vi "Apply Package Name to Enum Metadata.vi"(8 "error in":errorcluster, 10 "Package Name":string, 11 "gRPC Enum Metadata in":T1[](array[typedef])) -> (0 "error out":errorcluster, 3 "gRPC Enum Metadata out":T1[](array[typedef]))   [LabVIEW 2019, in "grpc-lvsupport.lvlib"]
uses:
  grpc-lvsupport.lvlib
  typeDefs/Enum Metadata.ctl
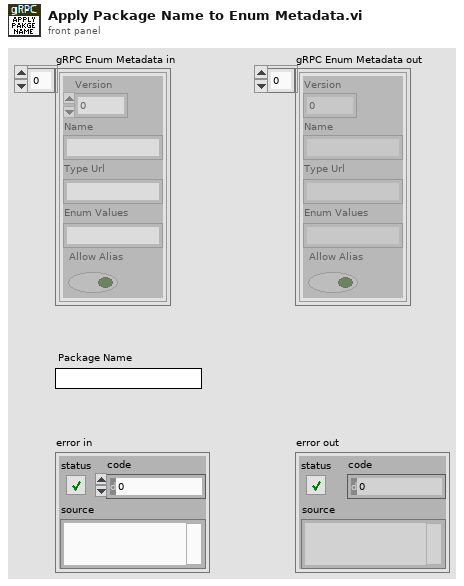
[diagram p1: front panel]
types:
  T1 = typedef "grpc-lvsupport.lvlib/Enum Metadata.ctl" = cluster{"Version":i32, "Name":string, "Type Url":string, "Enum Values":string, "Allow Alias":bool}
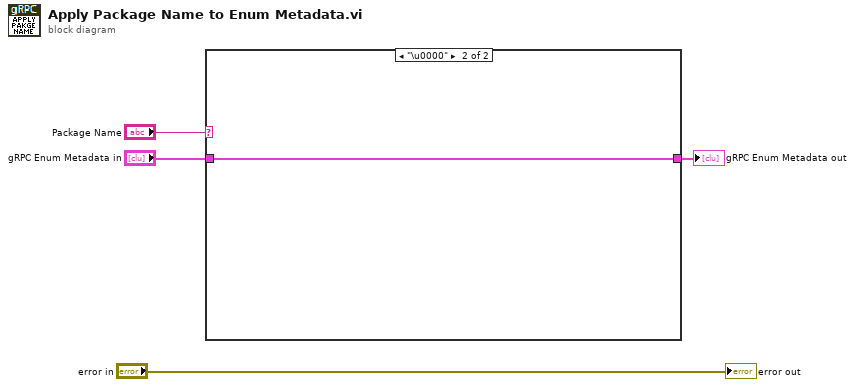
[diagram p0: block diagram]
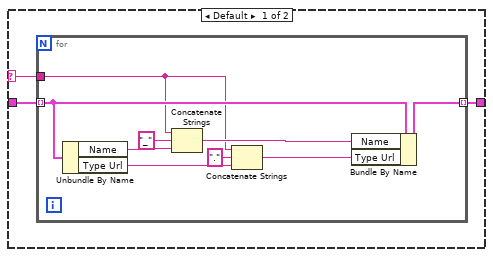
[diagram p2: hidden frame]
diagram:
  n1 = case shown="\"\"" "Package Name" {
    selector: "Package Name" -> [w5 _]
    tunnel: "gRPC Enum Metadata in" -> [w7 w17]
    tunnel: [w6 w17] -> w1
    frame Default {
      n2 = for {
        tunnel: w7 -> [w12] mode=indexing
        tunnel: w5 -> [w8]
        tunnel: [w9] -> w6 mode=indexing
        n3 = Unbundle By Name(w12) -> ("Name"=w16:string, "Type Url"=w13:string)
        n4 = Concatenate Strings(w8, "_" ("string"), w16) -> (w11:string)
        n5 = Concatenate Strings(w8, "." ("string"), w13) -> (w10:string)
        n6 = Bundle By Name(cluster=w12, "Name"=w11, "Type Url"=w10) -> (w9:T1)
      }
    }
    frame "\u0000" {
    }
  }
  "gRPC Enum Metadata out" <- w1
  "error out" <- "error in"
